vi "CNR abx MLE.vi"(0 "parameters":dbl[](array[numeric]), 1 "model function":T3, 9 "output control":T2={"model function"=TRUE, "gradient"=TRUE}, 11 "error in (no error)":errorcluster, 12 "Y":dbl[](array[numeric]), 13 "X":dbl[](array[numeric])) -> (2 "Jacobian":T1, 3 "number of function calls":i32, 4 "Hessian":T1, 6 "gradient":dbl[](array[numeric]), 8 "best fit":dbl[](array[numeric]), 10 "chiSqr":dbl, 15 "error out":errorcluster)   [LabVIEW 2021, in "Fits.lvlib"]
uses:
  Fits.lvlib
  <vilib>/Analysis/Matrix/Datatypes/RealMatrix.ctl
  <vilib>/gmath/NumericalOptimization/LM model function.ctl
  <vilib>/gmath/NumericalOptimization/LM model function reference.ctl
  <vilib>/gmath/NumericalOptimization/LM_output select.ctl
  <vilib>/Analysis/baseanly.llb/Real A x B.vi
  <vilib>/Analysis/baseanly.llb/A x Vector.vi
  <vilib>/gmath/NI_Gmath.lvlib
  <vilib>/Analysis/NI_AALBase.lvlib
  <vilib>/Analysis/Matrix/NI_Matrix.lvlib
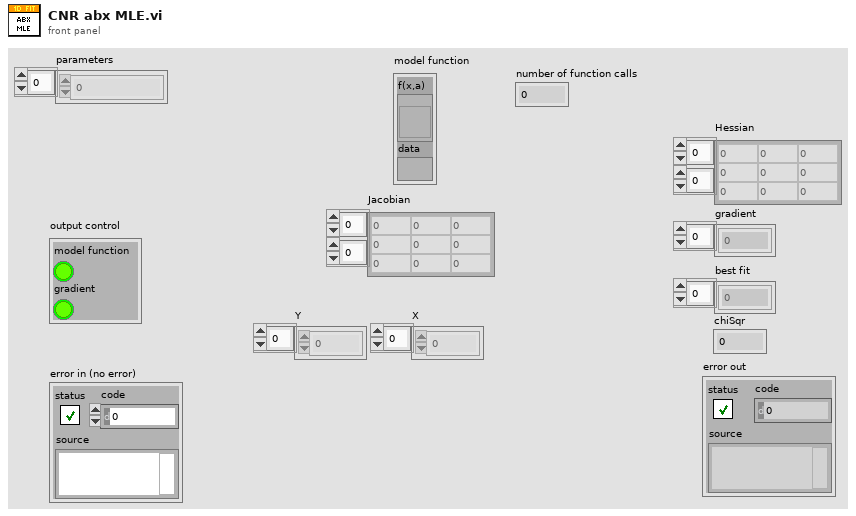
[diagram p1: front panel]
types:
  T1 = typedef "NI_Matrix.lvlib/RealMatrix.ctl" = dbl[][]
  T2 = typedef "NI_Gmath.lvlib/LM_output select.ctl" = cluster{"model function":bool, "gradient":bool}
  T3 = typedef "NI_Gmath.lvlib/LM model function.ctl" = cluster{"f(x,a)":T4, "data":variant}
  T4 = typedef "NI_Gmath.lvlib/LM model function reference.ctl" = refnum<vi>
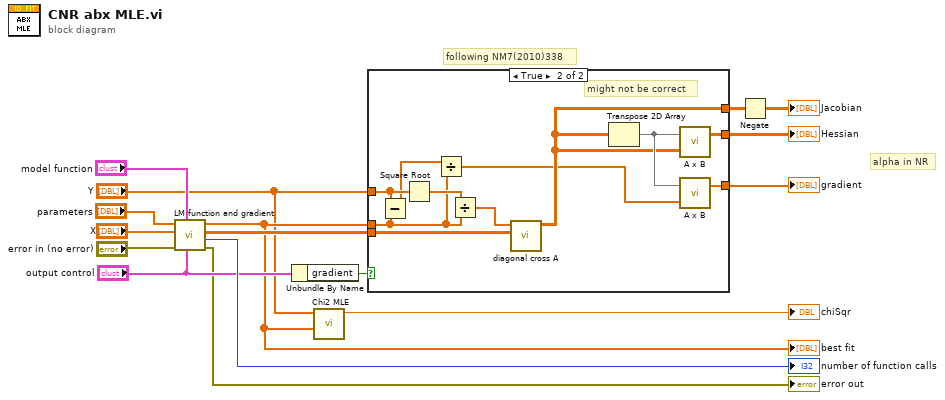
[diagram p0: block diagram]
diagram:
  # "alpha in NR"
  # "following NM7(2010)338"
  n1 = call <vilib>:"LM function and gradient.vi"("output control"="output control", "model function"="model function", "error in (no error)"="error in (no error)", "X"="X", "a"="parameters") -> ("error out"=→"error out":errorcluster, "number of function calls"=→"number of function calls":i32, "gradient"=w7:dbl[][], "f(X)"=w3:dbl[])  [unwired: 3 out]
  "best fit" <- w3
  n2 = Unbundle By Name("output control") -> ("gradient"=w13:bool)
  n3 = call "Chi2 MLE.vi"("f(X)"=w3, "Y"="Y") -> ("chi2_mle"=→"chiSqr":dbl)  [unwired: 9 in]
  n4 = case shown="True" w13 {
    tunnel: [_ w23] -> w11
    tunnel: [_ w24] -> w5
    tunnel: w7 -> [_ w27]
    tunnel: [_ w25] -> w6
    tunnel: w3 -> [_ w18]
    tunnel: "Y" -> [_ w20]
    frame False {
    }
    frame True {
      # "might not be correct"
      n5 = Subtract(x=w20, y=w18) -> (x-y=w19:dbl[])
      n6 = Square Root(x=w20) -> (sqrt(x)=w22:dbl[])
      n7 = Divide(x=w19, y=w18) -> (x/y=w17:dbl[])
      n8 = Divide(x=w22, y=w18) -> (x/y=w21:dbl[])
      n9 = call <vilib>:"diagonal cross A.vi"("A"=w27, "diagonal"=w21) -> ("diagonalxA"=w25:T1)  [unwired: 9 out]
      n10 = Transpose 2D Array(2D array=w25) -> (transposed array=w26:T1)
      n11 = call-poly <vilib>:"A x B.vi"("B"=w25, "A"=w26) -> ("A x B"=w24:T1)  [unwired: 1 out]
      n12 = call-poly <vilib>:"A x B.vi"("Vector"=w17, "A"=w26) -> ("A x Vector"=w23:dbl[])  [unwired: 1 out]
    }
  }
  "Hessian" <- w5
  "gradient" <- w11
  n13 = Negate(x=w6) -> (-x=→"Jacobian":T1)
